vi "Measure Scalar-Mixer Calibration Data.vi"(5 "Standard (0: Open)":u16(ring) items=["Open", "Short", "Load", "Thru", "Power Calibration"], 6 "Power Sensor (0:Power Sensor A)":u16(ring) items=["Power Sensor A", "Power Sensor B"], 7 "Channel (1)":i32=1, 8 "error in (no error)":errorcluster, 9 "Port 2 - specified freq. (1)":i32=1, 10 "Port 1 - measurement (1)":i32=1, 11 "VISA resource name":refnum<visa-resource-name>) -> (0 "error out":errorcluster, 3 "VISA resource name out":refnum<visa-resource-name>)   [LabVIEW 2020, in "Agilent ENA Series.lvlib"]
doc: "Measures the calibration data, for selected channel, of the open, short, load, thru standard or isolation of the specified ports.\n\n<b>Note:</b>\nThis VI is not supported by the E5063A, E5080A and E5080B."
uses:
  <instrlib>/Agilent ENA Series/Agilent ENA Series.lvlib
panel:
  # "Note:\nThis VI is not supported by the E5063A, E5080A and E5080B."
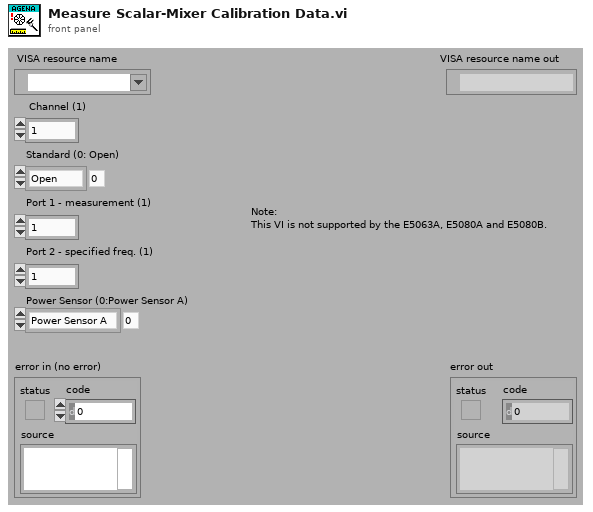
[diagram p1: front panel]
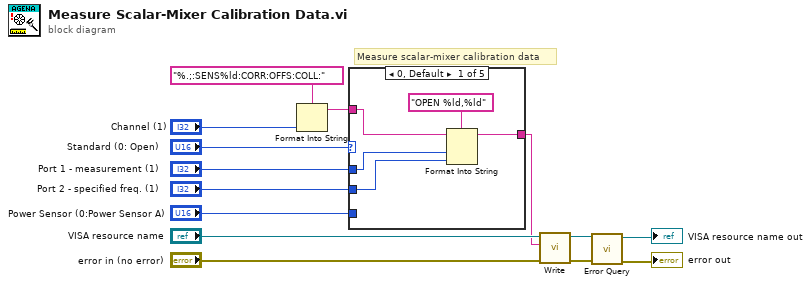
[diagram p0: block diagram]
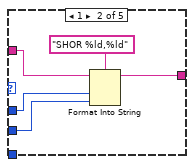
[diagram p2: hidden frame]
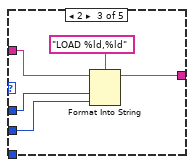
[diagram p3: hidden frame]
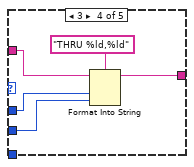
[diagram p4: hidden frame]
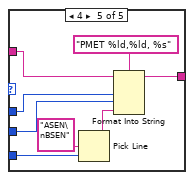
[diagram p5: hidden frame]
diagram:
  # "Measure scalar-mixer calibration data"
  n1 = Format Into String(format string="%.;:SENS%ld:CORR:OFFS:COLL:", "Channel (1)") -> (resulting string=w7:string)  [unwired: 2 in, 1 out]
  n2 = case shown="0, Default" "Standard (0: Open)" {
    tunnel: "Port 1 - measurement (1)" -> [w17 w22 w27 w32 w40]
    tunnel: "Port 2 - specified freq. (1)" -> [w15 w20 w25 w30 w38]
    tunnel: w7 -> [w18 w23 w28 w33 w41]
    tunnel: [w16 w21 w26 w31 w39] -> w6
    tunnel: "Power Sensor (0:Power Sensor A)" -> [_ _ _ _ w36]
    frame 0, Default {
      n3 = Format Into String(format string="OPEN %ld,%ld", initial string=w18, w17, w15) -> (resulting string=w16:string)  [unwired: 1 in, 1 out]
    }
    frame 1 {
      n4 = Format Into String(format string="SHOR %ld,%ld", initial string=w23, w22, w20) -> (resulting string=w21:string)  [unwired: 1 in, 1 out]
    }
    frame 2 {
      n5 = Format Into String(format string="LOAD %ld,%ld", initial string=w28, w27, w25) -> (resulting string=w26:string)  [unwired: 1 in, 1 out]
    }
    frame 3 {
      n6 = Format Into String(format string="THRU %ld,%ld", initial string=w33, w32, w30) -> (resulting string=w31:string)  [unwired: 1 in, 1 out]
    }
    frame 4 {
      n7 = Pick Line(multi-line string="ASEN\nBSEN", line index=w36) -> (output string=w35:string)  [unwired: 1 in]
      n8 = Format Into String(format string="PMET %ld,%ld, %s", initial string=w41, w40, w38, w35) -> (resulting string=w39:string)  [unwired: 1 in, 1 out]
    }
  }
  n9 = call <instrlib>:"Write.vi"("error in (no error)"="error in (no error)", "String ()"=w6, "VISA resource name"="VISA resource name") -> ("error out"=w3:errorcluster, "VISA resource name out"=w4:refnum<visa-resource-name>)  [unwired: 6 in, 1 out]
  n10 = call <instrlib>:"Error Query.vi"("error in (no error)"=w3, "VISA resource name"=w4) -> ("error out"=→"error out":errorcluster, "VISA resource name out"=→"VISA resource name out":refnum<visa-resource-name>)  [unwired: 6 in, 2 out]
